vi "Esophageal_Datalogger_PauseButton.vi"(8 "error in (no error)":errorcluster, 11 "Log File In":refnum<file>) -> (0 "error out":errorcluster, 3 "Log File Out":refnum<file>)   [LabVIEW 2021]
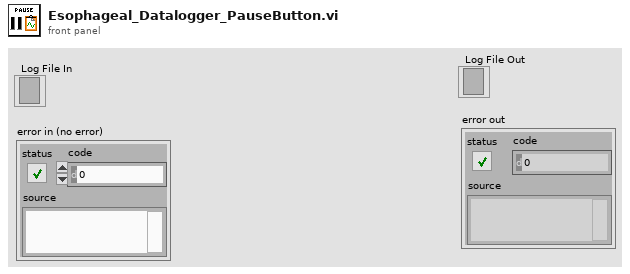
[diagram p1: front panel]
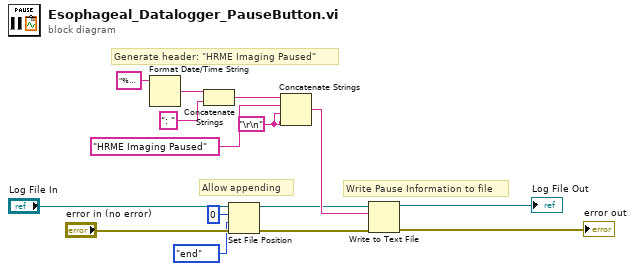
[diagram p0: block diagram]
diagram:
  w3 = "\r\n"
  # "Write Pause Information to file"
  # "Generate header: \"HRME Imaging Paused\""
  # "Allow appending"
  n1 = Format Date/Time String(time format string (%c)="%H%M%S%3u") -> (date/time string=w10:string)  [unwired: 2 in]
  n2 = Concatenate Strings(w10, ": " ("string")) -> (w12:string)
  n3 = Set File Position(offset (in bytes) (0)=i64 0, refnum="Log File In", from (0:start)=enum16{"start", "end", "current"}."end", error in="error in (no error)") -> (refnum out=w8:refnum<file>, error out=w15:errorcluster)
  n4 = Concatenate Strings(w12, "HRME Imaging Paused" ("time format string (%c)"), w3, w3) -> (w14:string)
  n5 = Write to Text File(file (use dialog)=w8, text=w14, error in=w15) -> (refnum out=→"Log File Out":refnum<file>, error out=→"error out":errorcluster)  [unwired: 1 in, 1 out]
